vi "Is Root.vi"(11 "Module in":refnum<class "Module.lvclass">) -> (2 "Is Root":bool, 3 "Module out":refnum<class "Module.lvclass">)   [LabVIEW 2020, in "Volatus.lvlib" / "Module.lvclass"]
uses:
  Module.lvclass
  Module.lvclass/Module.ctl
  MessageQ/MessageQ.lvclass
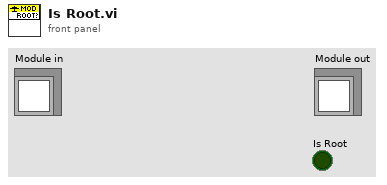
[diagram p1: front panel]
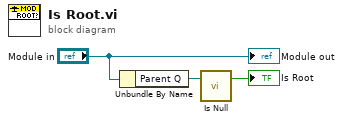
[diagram p0: block diagram]
diagram:
  n1 = Unbundle By Name("Module in") -> ("Parent Q"=w2:refnum<class "MessageQ.lvclass">)
  n2 = call "Is Null.vi"("MessageQ in"=w2) -> ("Null"=→"Is Root":bool)  [unwired: 2 in]
  "Module out" <- "Module in"
